vi "LVClass_SlopesPostProcessList AddProcessorTabWithVaraint.vi"(0 "SlopesPostProcessorList in":refnum<class "SlopesPostProcessorList.lvclass">, 7 "Processing list in":T1[](array[typedef]), 9 "Enum":enum16{"As new list", "Append", "InsertFront"}(ring), 11 "error in":errorcluster) -> (4 "SlopesPostProcessorList out":refnum<class "SlopesPostProcessorList.lvclass">, 15 "error out":errorcluster)   [LabVIEW 2020, in "SlopesPostProcessorList.lvclass"]
uses:
  SlopesPostProcessorList.lvclass
  Controls/SlopesPostProcessorList - ONE - with variant.ctl
  Controls/SlopesStructToVariant.ctl
  Controls/Point2D.ctl
  Controls/Point2Df.ctl
  Controls/Slopes origin - SlopesPostProcessingList.ctl
  HasoSlopes/HasoSlopes.lvclass
  Controls/PupillStructToVariant.ctl
  Controls/General dimensions definition.ctl
  Pupil/Pupil.lvclass
  Controls/SlopesPostProcessorList - Double passage.ctl
  Controls/SlopesPostProcessorList - Filter.ctl
  Controls/SlopesPostProcessorList - Modulator.ctl
  Controls/SlopesPostProcessorList - Add lens.ctl
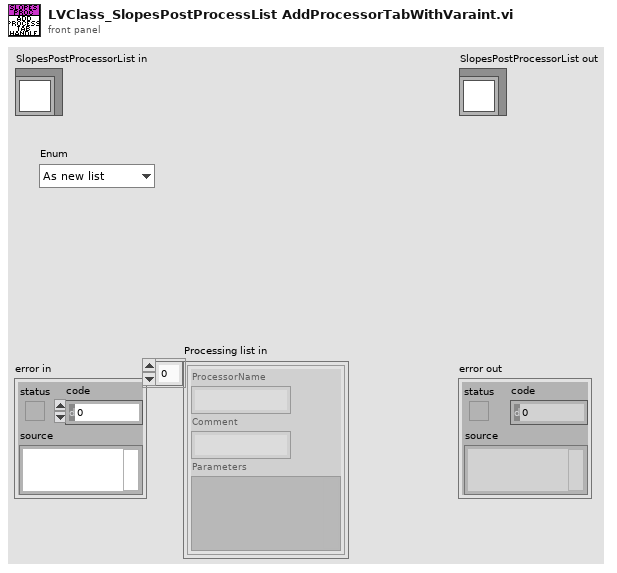
[diagram p1: front panel]
types:
  T1 = typedef "SlopesPostProcessorList - ONE - with variant.ctl" = cluster{"ProcessorName":string, "Comment":string, "Parameters":variant}
  T2 = typedef "SlopesPostProcessorList - Double passage.ctl" = cluster{"ActivateOnTilt":bool, "ActivateOnCurvature":bool}
  T3 = typedef "SlopesPostProcessorList - Filter.ctl" = cluster{"tiltx":bool, "tilty":bool, "curv":bool, "astig0":bool, "astig45":bool, "others":bool}
  T4 = typedef "SlopesPostProcessorList - Modulator.ctl" = cluster{"tiltx":sgl, "tilty":sgl, "curv":sgl, "astig0":sgl, "astig45":sgl, "others":sgl}
  T5 = typedef "SlopesPostProcessorList - Add lens.ctl" = cluster{"lens_m":sgl, "KeepCurvature":bool}
  T6 = typedef "SlopesStructToVariant.ctl" = cluster{"dimension":cluster{"size":T7, "step":T8}, "HASO serial number":string, "REF Type":T9, "Slopes from XML string format":string}
  T7 = typedef "Point2D.ctl" = cluster{"X":u32, "Y":u32}
  T8 = typedef "Point2Df.ctl" = cluster{"X":sgl, "Y":sgl}
  T9 = typedef "Slopes origin - SlopesPostProcessingList.ctl" = enum16{"Slopes from acq", "Slopes from file", "Slopes from data"}
  T10 = typedef "PupillStructToVariant.ctl" = cluster{"Dimension":T11, "Data":i32[][]}
  T11 = typedef "General dimensions definition.ctl" = cluster{"Size":T7, "Step":T8}
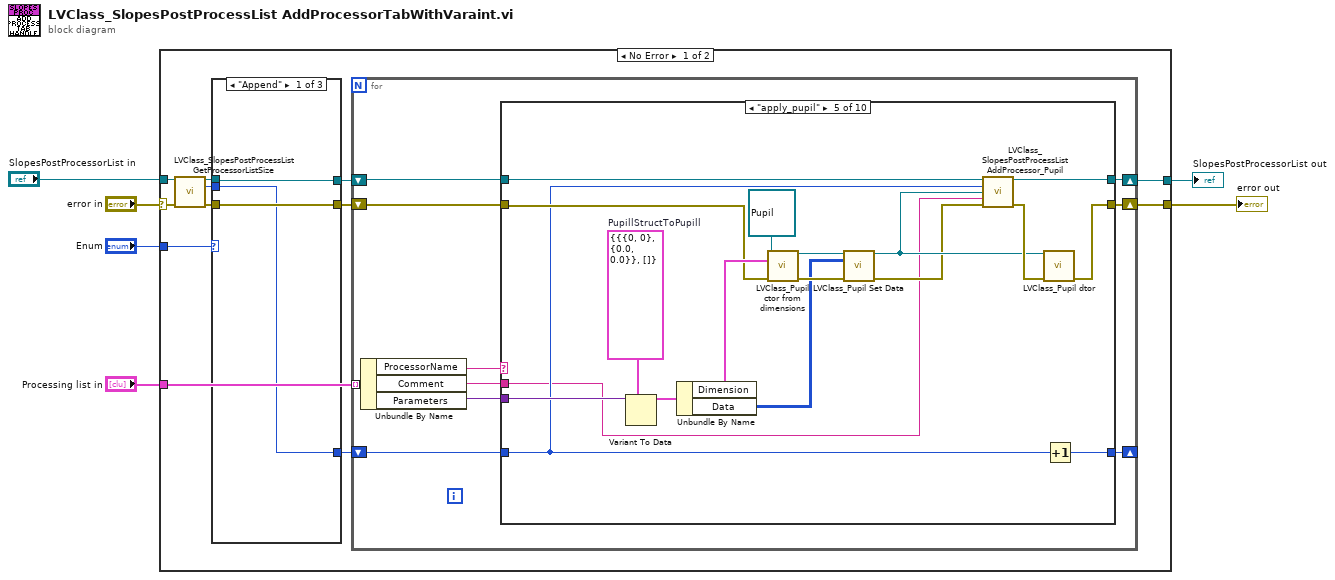
[diagram p0: block diagram]
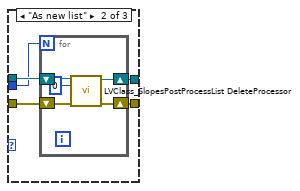
[diagram p2: hidden frame]
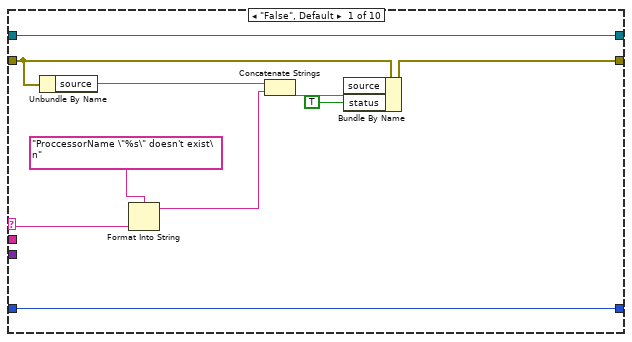
[diagram p4: hidden frame]
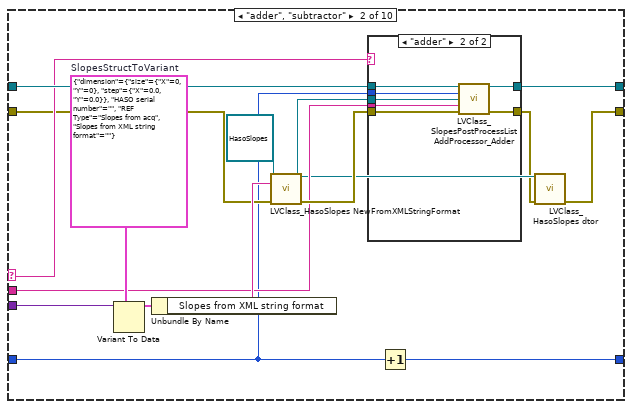
[diagram p5: hidden frame]
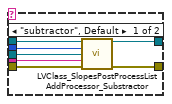
[diagram p6: hidden frame]
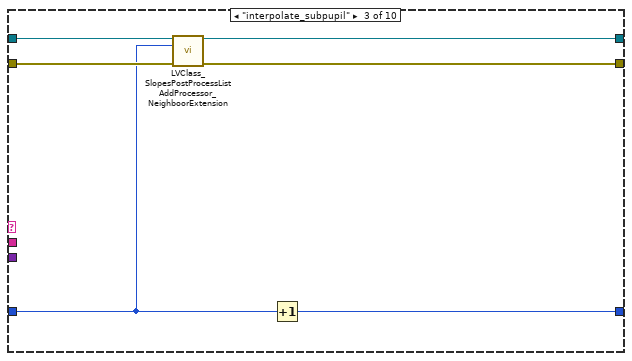
[diagram p7: hidden frame]
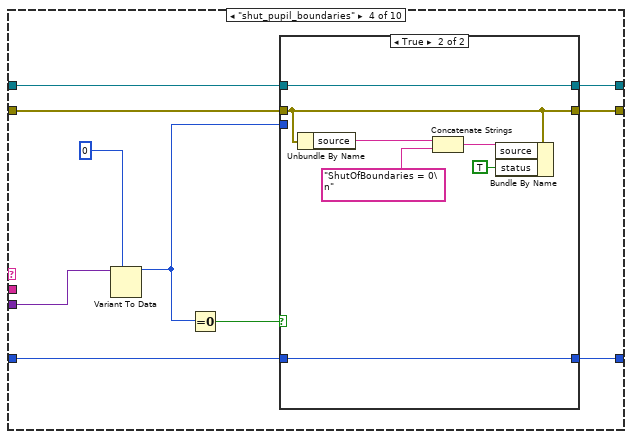
[diagram p8: hidden frame]
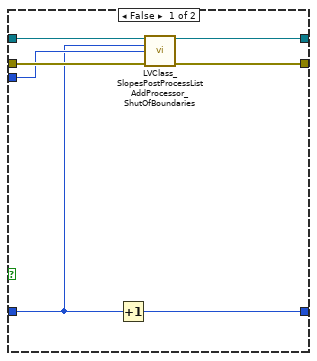
[diagram p9: hidden frame]
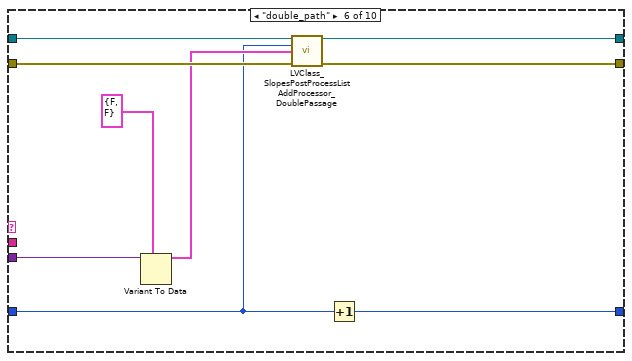
[diagram p10: hidden frame]
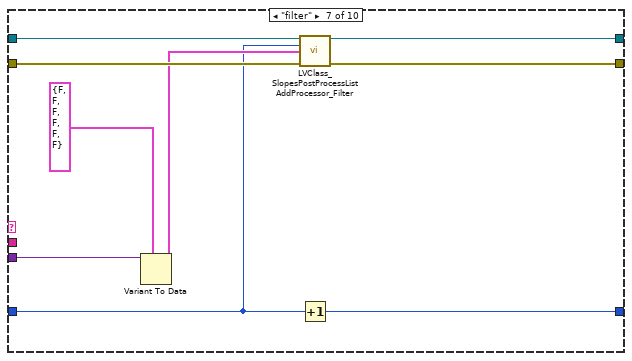
[diagram p11: hidden frame]
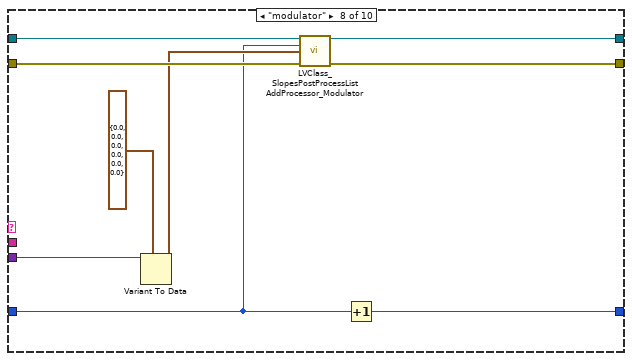
[diagram p12: hidden frame]
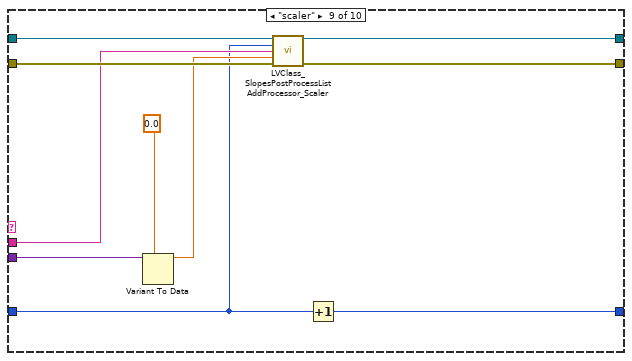
[diagram p13: hidden frame]
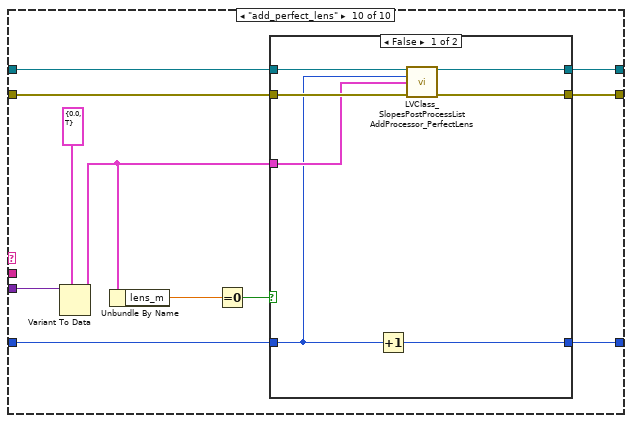
[diagram p14: hidden frame]
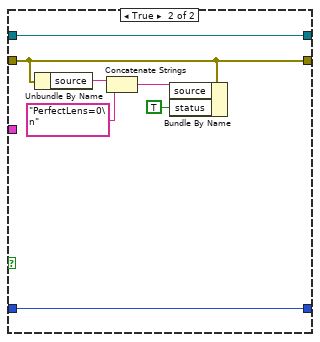
[diagram p15: hidden frame]
diagram:
  n1 = case shown="No Error" "error in" {
    selector: "error in" -> [w15 w195]
    tunnel: [w16 w195] -> w5
    tunnel: [w17 w194] -> w6
    tunnel: "SlopesPostProcessorList in" -> [w14 w194]
    tunnel: "Processing list in" -> [w18 _]
    tunnel: "Enum" -> [w9 _]
    frame No Error {
      n2 = call "LVClass_SlopesPostProcessList GetProcessorListSize.vi"("SlopesPostProcessorList in"=w14, "error in (no error)"=w15) -> ("SlopesPostProcessorList out"=w13:refnum<class "SlopesPostProcessorList.lvclass">, "size"=w8:u32, "error out"=w11:errorcluster)  [unwired: 11 in]
      n3 = case shown="\"Append\"" w9 {
        tunnel: w13 -> [w21 w26 w33]
        tunnel: [w21 w25 w33] -> w12
        tunnel: w11 -> [w20 w24 w32]
        tunnel: [w20 w23 w32] -> w10
        tunnel: w8 -> [w19 w22 _]
        tunnel: [w19 _ _] -> w7
        frame "Append" {
        }
        frame "As new list" {
          n4 = for {
            N: w22 -> [_]
            shift-right: [w30] -> w25
            shift-left: w26 -> [w31]
            shift-right: [w28] -> w23
            shift-left: w24 -> [w29]
            n5 = call "LVClass_SlopesPostProcessList DeleteProcessor.vi"("SlopesPostProcessorList in"=w31, "Position"=0, "error in (no error)"=w29) -> ("SlopesPostProcessorList out"=w30:refnum<class "SlopesPostProcessorList.lvclass">, "error out"=w28:errorcluster)  [unwired: 11 in]
          }
        }
        frame "InsertFront" {
        }
      }
      n6 = for {
        tunnel: w18 -> [w37] mode=indexing
        shift-right: [w41] -> w16
        shift-left: w10 -> [w42]
        shift-right: [w39] -> w17
        shift-left: w12 -> [w40]
        shift-right: [w35] -> _
        shift-left: w7 -> [w34]
        n7 = Unbundle By Name(w37) -> ("ProcessorName"=w43:string, "Comment"=w36:string, "Parameters"=w38:variant)
        n8 = case shown="\"apply_pupil\"" w43 {
          selector: w43 -> [w46 w67 _ _ _ _ _ _ _ _]
          tunnel: w42 -> [w53 w61 w87 w98 w119 w138 w147 w156 w166 w178]
          tunnel: [w45 w56 w86 w97 w126 w137 w145 w154 w165 w179] -> w41
          tunnel: w34 -> [w44 w55 w85 w94 w116 w133 w142 w151 w160 w174]
          tunnel: w40 -> [w47 w69 w89 w96 w130 w140 w148 w157 w168 w176]
          tunnel: [w47 w68 w88 w95 w131 w139 w146 w155 w167 w175] -> w39
          tunnel: w38 -> [_ w65 _ w91 w128 w135 w149 w158 w162 w173]
          tunnel: w36 -> [_ w59 _ _ w114 _ _ _ w164 _]
          tunnel: [w44 w54 w84 w90 w115 w132 w141 w150 w159 w169] -> w35
          frame "False", Default {
            n9 = Unbundle By Name(w53) -> ("source"=w51:string)
            n10 = Format Into String(format string="ProccessorName \"%s\" doesn't exist\n" ("source"), w46) -> (resulting string=w49:string)  [unwired: 2 in, 1 out]
            n11 = Concatenate Strings(w51, w49) -> (w50:string)
            n12 = Bundle By Name(cluster=w53, "source"=w50, "status"=TRUE) -> (w45:errorcluster)
          }
          frame "adder", "subtractor" {
            w66 = T6 {"dimension"={"size"={"X"=0, "Y"=0}, "step"={"X"=0.0, "Y"=0.0}}, "HASO serial number"="", "REF Type"=enum."Slopes from acq", "Slopes from XML string format"=""}  # SlopesStructToVariant
            n13 = Variant To Data(type=w66, Variant=w65) -> (data=w64:T6)  [unwired: 1 in, 1 out]
            n14 = Unbundle By Name(w64) -> ("Slopes from XML string format"=w63:string)
            n15 = call "LVClass_HasoSlopes NewFromXMLStringFormat.vi"("HasoSlopes in"=refnum<class "HasoSlopes.lvclass"> refnum, "XML txt format"=w63, "error in (no error)"=w61) -> ("HasoSlopes out"=w58:refnum<class "HasoSlopes.lvclass">, "error out"=w60:errorcluster)  [unwired: 11 in]
            n16 = case shown="\"adder\"" w67 {
              tunnel: w69 -> [w76 w83]
              tunnel: [w71 w82] -> w68
              tunnel: w55 -> [w75 w81]
              tunnel: w59 -> [w73 w80]
              tunnel: w58 -> [w74 w79]
              tunnel: w60 -> [w72 w78]
              tunnel: [w70 w77] -> w57
              frame "subtractor", Default {
                n17 = call "LVClass_SlopesPostProcessList AddProcessor_Substractor.vi"("SlopesPostProcessorList in"=w76, "Position"=w75, "HasoSlopes.lvclass"=w74, "Comment"=w73, "error in (no error)"=w72) -> ("SlopesPostProcessorList out"=w71:refnum<class "SlopesPostProcessorList.lvclass">, "error out"=w70:errorcluster)  [unwired: 9 in]
              }
              frame "adder" {
                n18 = call "LVClass_SlopesPostProcessList AddProcessor_Adder.vi"("SlopesPostProcessorList in"=w83, "Position"=w81, "HasoSlopes.lvclass"=w79, "Comment"=w80, "error in (no error)"=w78) -> ("SlopesPostProcessorList out"=w82:refnum<class "SlopesPostProcessorList.lvclass">, "error out"=w77:errorcluster)  [unwired: 9 in]
              }
            }
            n19 = Increment(x=w55) -> (x+1=w54:u32)
            n20 = call "LVClass_HasoSlopes dtor.vi"("HasoSlopes in"=w58, "error in (no error)"=w57) -> ("error out"=w56:errorcluster)  [unwired: 12 in, 1 out]
          }
          frame "interpolate_subpupil" {
            n21 = call "LVClass_SlopesPostProcessList AddProcessor_NeighboorExtension.vi"("SlopesPostProcessorList in"=w89, "Position"=w85, "error in (no error)"=w87) -> ("SlopesPostProcessorList out"=w88:refnum<class "SlopesPostProcessorList.lvclass">, "error out"=w86:errorcluster)  [unwired: 11 in]
            n22 = Increment(x=w85) -> (x+1=w84:u32)
          }
          frame "shut_pupil_boundaries" {
            n23 = Variant To Data(type=u32 0 ("ShutOfBoundaries"), Variant=w91) -> (data=w92:u32)  [unwired: 1 in, 1 out]
            n24 = Equal To 0?(x=w92) -> (x = 0?=w99:bool)
            n25 = case shown="True" w99 {
              tunnel: w98 -> [w105 w107]
              tunnel: [w104 w107] -> w97
              tunnel: w96 -> [w106 w109]
              tunnel: [w103 w109] -> w95
              tunnel: w94 -> [w101 w108]
              tunnel: w92 -> [w102 _]
              tunnel: [w100 w108] -> w90
              frame False {
                n26 = Increment(x=w101) -> (x+1=w100:u32)
                n27 = call "LVClass_SlopesPostProcessList AddProcessor_ShutOfBoundaries.vi"("SlopesPostProcessorList in"=w106, "Position"=w101, "ShutOfBoundaries"=w102, "error in (no error)"=w105) -> ("SlopesPostProcessorList out"=w103:refnum<class "SlopesPostProcessorList.lvclass">, "error out"=w104:errorcluster)  [unwired: 10 in]
              }
              frame True {
                n28 = Unbundle By Name(w107) -> ("source"=w112:string)
                n29 = Concatenate Strings(w112, "ShutOfBoundaries = 0\n" ("source")) -> (w111:string)
                n30 = Bundle By Name(cluster=w107, "source"=w111, "status"=TRUE) -> ()  [unwired: 1 out]
              }
            }
          }
          frame "apply_pupil" {
            w129 = T10 {"Dimension"={"Size"={"X"=0, "Y"=0}, "Step"={"X"=0.0, "Y"=0.0}}, "Data"=[]}  # PupillStructToPupill
            n31 = Variant To Data(type=w129, Variant=w128) -> (data=w121:T10)  [unwired: 1 in, 1 out]
            n32 = Unbundle By Name(w121) -> ("Dimension"=w120:T11, "Data"=w117:i32[][])
            n33 = call "LVClass_Pupil ctor from dimensions.vi"("Pupil (const)"=refnum<class "Pupil.lvclass"> refnum ("Pupil in"), "Dimensions_um"=w120, "error in (no error)"=w119) -> ("Pupil (new)"=w122:refnum<class "Pupil.lvclass">, "error out"=w123:errorcluster)  [unwired: 11 in]
            n34 = call "LVClass_Pupil Set Data.vi"("Pupil in"=w122, "Data"=w117, "error in (no error)"=w123) -> ("Pupil out"=w125:refnum<class "Pupil.lvclass">, "error out"=w124:errorcluster)  [unwired: 11 in]
            n35 = call "LVClass_SlopesPostProcessList AddProcessor_Pupil.vi"("SlopesPostProcessorList in"=w130, "Position"=w116, "Pupil.lvclass"=w125, "Comment"=w114, "error in (no error)"=w124) -> ("SlopesPostProcessorList out"=w131:refnum<class "SlopesPostProcessorList.lvclass">, "error out"=w127:errorcluster)  [unwired: 9 in]
            n36 = call "LVClass_Pupil dtor.vi"("Pupil in"=w125, "error in (no error)"=w127) -> ("error out"=w126:errorcluster)  [unwired: 12 in, 1 out]
            n37 = Increment(x=w116) -> (x+1=w115:u32)
          }
          frame "double_path" {
            n38 = Variant To Data(type=T2 {"ActivateOnTilt"=FALSE, "ActivateOnCurvature"=FALSE} ("doublePassage"), Variant=w135) -> (data=w134:T2)  [unwired: 1 in, 1 out]
            n39 = call "LVClass_SlopesPostProcessList AddProcessor_DoublePassage.vi"("SlopesPostProcessorList in"=w140, "Position"=w133, "doublePath"=w134, "error in (no error)"=w138) -> ("SlopesPostProcessorList out"=w139:refnum<class "SlopesPostProcessorList.lvclass">, "error out"=w137:errorcluster)  [unwired: 10 in]
            n40 = Increment(x=w133) -> (x+1=w132:u32)
          }
          frame "filter" {
            n41 = Variant To Data(type=T3 {"tiltx"=FALSE, "tilty"=FALSE, "curv"=FALSE, "astig0"=FALSE, "astig45"=FALSE, "others"=FALSE} ("Filter"), Variant=w149) -> (data=w143:T3)  [unwired: 1 in, 1 out]
            n42 = call "LVClass_SlopesPostProcessList AddProcessor_Filter.vi"("SlopesPostProcessorList in"=w148, "Position"=w142, "Filter"=w143, "error in (no error)"=w147) -> ("SlopesPostProcessorList out"=w146:refnum<class "SlopesPostProcessorList.lvclass">, "error out"=w145:errorcluster)  [unwired: 10 in]
            n43 = Increment(x=w142) -> (x+1=w141:u32)
          }
          frame "modulator" {
            n44 = Variant To Data(type=T4 {"tiltx"=0.0, "tilty"=0.0, "curv"=0.0, "astig0"=0.0, "astig45"=0.0, "others"=0.0} ("Modulator"), Variant=w158) -> (data=w152:T4)  [unwired: 1 in, 1 out]
            n45 = call "LVClass_SlopesPostProcessList AddProcessor_Modulator.vi"("SlopesPostProcessorList in"=w157, "Position"=w151, "Modulator"=w152, "error in (no error)"=w156) -> ("SlopesPostProcessorList out"=w155:refnum<class "SlopesPostProcessorList.lvclass">, "error out"=w154:errorcluster)  [unwired: 10 in]
            n46 = Increment(x=w151) -> (x+1=w150:u32)
          }
          frame "scaler" {
            n47 = Variant To Data(type=sgl 0.0 ("scaler"), Variant=w162) -> (data=w161:sgl)  [unwired: 1 in, 1 out]
            n48 = call "LVClass_SlopesPostProcessList AddProcessor_Scaler.vi"("SlopesPostProcessorList in"=w168, "Position"=w160, "comment"=w164, "scaler"=w161, "error in (no error)"=w166) -> ("SlopesPostProcessorList out"=w167:refnum<class "SlopesPostProcessorList.lvclass">, "error out"=w165:errorcluster)  [unwired: 9 in]
            n49 = Increment(x=w160) -> (x+1=w159:u32)
          }
          frame "add_perfect_lens" {
            n50 = Variant To Data(type=T5 {"lens_m"=0.0, "KeepCurvature"=TRUE} ("Perfect lens"), Variant=w173) -> (data=w171:T5)  [unwired: 1 in, 1 out]
            n51 = Unbundle By Name(w171) -> ("lens_m"=w177:sgl)
            n52 = Equal To 0?(x=w177) -> (x = 0?=w170:bool)
            n53 = case shown="False" w170 {
              tunnel: w178 -> [w183 w187]
              tunnel: [w184 w187] -> w179
              tunnel: w176 -> [w186 w189]
              tunnel: [w185 w189] -> w175
              tunnel: w174 -> [w181 w188]
              tunnel: w171 -> [w182 _]
              tunnel: [w180 w188] -> w169
              frame False {
                n54 = Increment(x=w181) -> (x+1=w180:u32)
                n55 = call "LVClass_SlopesPostProcessList AddProcessor_PerfectLens.vi"("SlopesPostProcessorList in"=w186, "Position"=w181, "Perfect lens"=w182, "error in (no error)"=w183) -> ("SlopesPostProcessorList out"=w185:refnum<class "SlopesPostProcessorList.lvclass">, "error out"=w184:errorcluster)  [unwired: 10 in]
              }
              frame True {
                n56 = Unbundle By Name(w187) -> ("source"=w192:string)
                n57 = Concatenate Strings(w192, "PerfectLens=0\n" ("source")) -> (w191:string)
                n58 = Bundle By Name(cluster=w187, "source"=w191, "status"=TRUE) -> ()  [unwired: 1 out]
              }
            }
          }
        }
      }
    }
    frame Error {
    }
  }
  "error out" <- w5
  "SlopesPostProcessorList out" <- w6
